vi "Syslog Device Example.vi"() -> ()   [LabVIEW 2016, in "Logger.syslog.lvclass"]
doc: "This VI illustrates sending Syslog debug messages to a collector using the Syslog reference design library."
uses:
  Logger.syslog.lvclass
  <userlib>/_SEH/Controls/CEH/CEH Actions.ctl
  <vilib>/NI/syslog/_subVIs/TypeDefs/syslog_severity_codes.ctl
  <vilib>/NI/syslog/_subVIs/TypeDefs/syslog_facility_codes.ctl
  <userlib>/_OpenG.lib/numeric/numeric.llb/Random Number Within Range - DBL__ogtk.vi
panel:
  out "Waveform Chart":dbl(graph)
  out "Syslog Messages Sent":string
  in  "Collector IP Address":string="0.0.0.0"
  in  "stop":bool
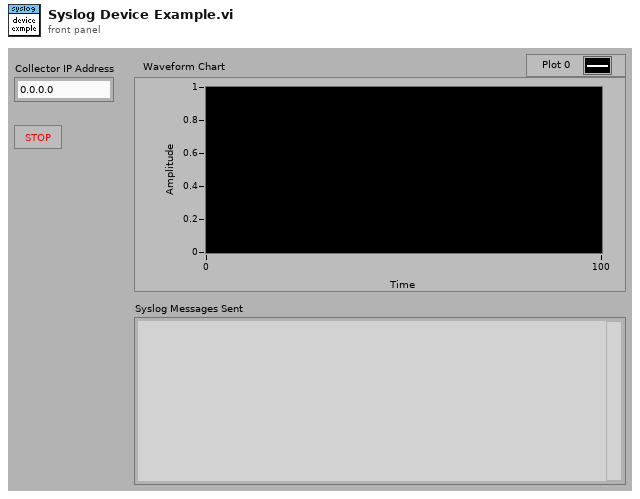
[diagram p1: front panel]
types:
  T1 = typedef "syslog_facility_codes.ctl" = enum16{"kernel", "user", "mail", "system daemons", "security/authorization", "syslogd", "line printer", "network news", "uucp", "clock daemon", "security/authorization (alternate)", "FTP daemon", "NTP subsystem", "log audit", "log alert", "clock daemon (alternate)", "local use 0", "local use 1", "local use 2", "local use 3", "local use 4", "local use 5", "local use 6", "local use 7"}
  T2 = typedef "syslog_severity_codes.ctl" = enum16{"emergency", "alert", "critical", "error", "warning", "notice", "info", "debug"}
  T3 = typedef "CEH Actions.ctl" = enum16{"Log", "Display Error Message", "Safe State", "Shutdown"}
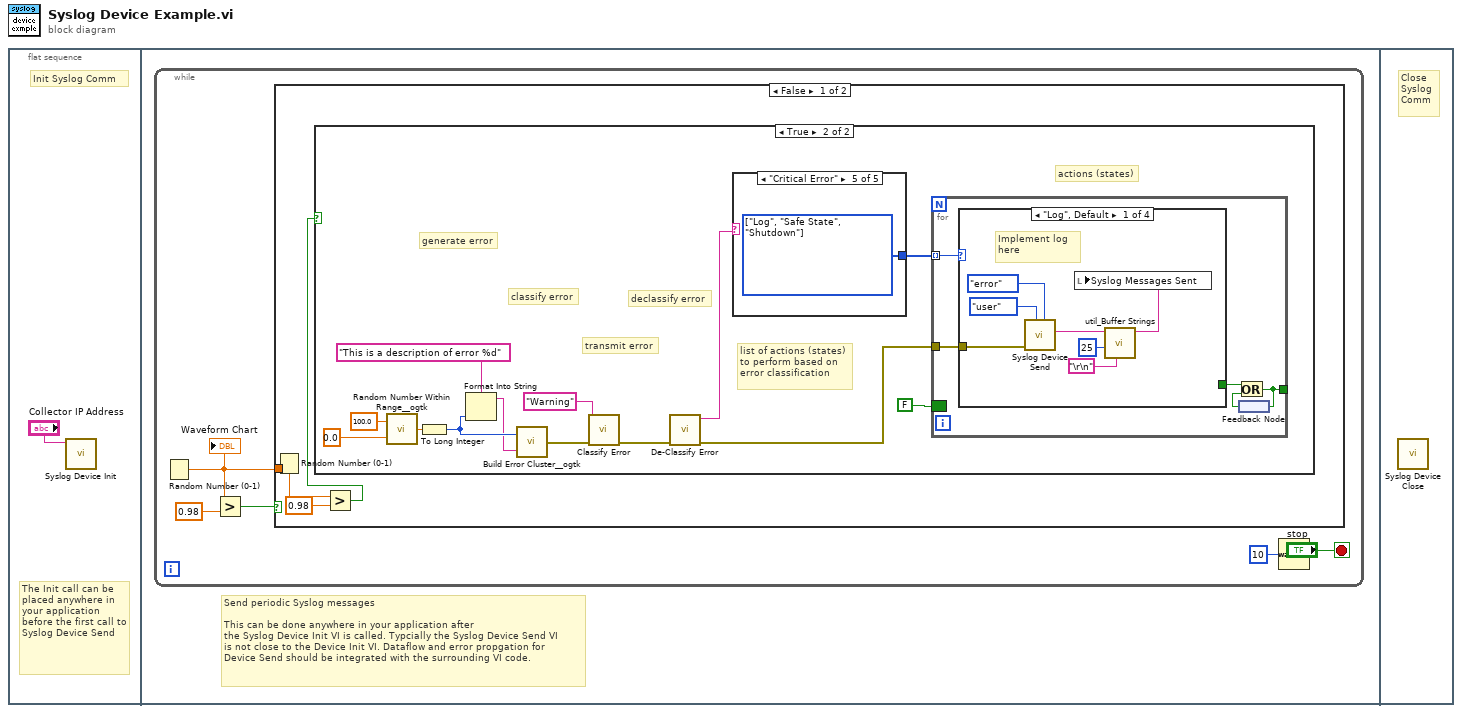
[diagram p0: block diagram]
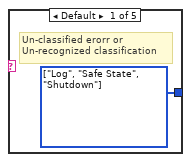
[diagram p3: hidden frame]
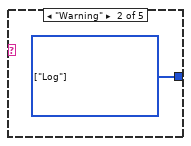
[diagram p4: hidden frame]
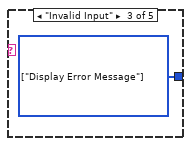
[diagram p5: hidden frame]
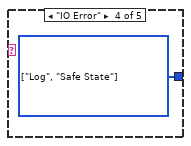
[diagram p6: hidden frame]
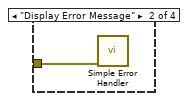
[diagram p7: hidden frame]
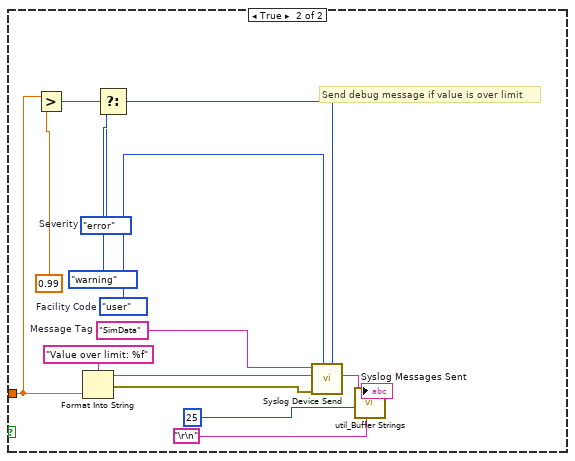
[diagram p10: hidden frame]
diagram:
  n1 = flat-sequence {
    frame #0 {
      # "The Init call can be placed anywhere in your application before the first call to Syslog Device Send"
      # "Init Syslog Comm"
      n2 = call <vilib>:"Syslog Device Init.vi"("Syslog Collector IP Address"="Collector IP Address") -> ()  [unwired: 10 in, 1 out]
    }
    frame #1 {
      # "Send periodic Syslog messages\n\nThis can be done anywhere in your application after\nthe Syslog Device Init VI is called. Typcially the Syslog Device Send VI\nis not close to the Device Init VI. Dataflow and error propgation for \nDevice Send should be integrated with the surrounding VI code."
      n3 = while {
        stop <- "stop" stop-if-true
        n4 = Random Number (0-1)() -> (number: 0 to 1=w2:dbl)
        "Waveform Chart" <- w2
        n5 = Greater?(x=w2, y=0.98) -> (0:w3:bool)
        n6 = case shown="False" w3 {
          tunnel: w2 -> [_ w53]
          frame False {
            n7 = Random Number (0-1)() -> (number: 0 to 1=w9:dbl)
            n8 = Greater?(x=w9, y=0.98) -> (0:w7:bool)
            n9 = case shown="True" w7 {
              frame False {
              }
              frame True {
                # "actions (states)"
                # "list of actions (states)\nto perform based on\nerror classification"
                # "declassify error"
                # "transmit error"
                # "classify error"
                # "generate error"
                n10 = call-poly <userlib>:"Random Number Within Range__ogtk.vi"("High"=100.0, "Low"=0.0) -> ("Random Number"=w19:dbl)  [unwired: 3 in]
                n11 = To Long Integer(number=w19) -> (32bit integer=w18:i32)
                n12 = Format Into String(format string="This is a description of error %d" ("String to Prepend to source (\"\")"), w18) -> (resulting string=w16:string)  [unwired: 2 in, 1 out]
                n13 = call <userlib>:"Build Error Cluster__ogtk.vi"("String to Prepend to source (\"\")"=w16, "code"=w18) -> ("error out"=w17:errorcluster)
                n14 = call <userlib>:"Classify Error.vi"("Error to Classify"=w17, "String"="Warning") -> ("Classified Error"=w13:errorcluster)  [unwired: 9 in]
                n15 = call <userlib>:"De-Classify Error.vi"("Classified Error"=w13) -> ("De-Classified Error"=w10:errorcluster, "Error Classification"=w12:string)  [unwired: 8 in, 1 out]
                n16 = case shown="\"Critical Error\"" w12 {
                  tunnel: [w23 w24 w25 w26 w27] -> w11
                  frame Default {
                    w23 = T3[] [enum."Log", enum."Safe State", enum."Shutdown"] items=["Log", "Display Error Message", "Safe State", "Shutdown"]
                    # "Un-classified erorr or\nUn-recognized classification"
                  }
                  frame "Warning" {
                    w24 = T3[] [enum."Log"] items=["Log", "Display Error Message", "Safe State", "Shutdown"]
                  }
                  frame "Invalid Input" {
                    w25 = T3[] [enum."Display Error Message"] items=["Log", "Display Error Message", "Safe State", "Shutdown"]
                  }
                  frame "IO Error" {
                    w26 = T3[] [enum."Log", enum."Safe State"] items=["Log", "Display Error Message", "Safe State", "Shutdown"]
                  }
                  frame "Critical Error" {
                    w27 = T3[] [enum."Log", enum."Safe State", enum."Shutdown"] items=["Log", "Display Error Message", "Safe State", "Shutdown"]
                  }
                }
                n17 = for {
                  tunnel: w10 -> [w31]
                  tunnel: w11 -> [w32] mode=indexing
                  border: FALSE -> [_]
                  tunnel: [w28] -> _
                  n18 = case shown="\"Log\", Default" w32 {
                    tunnel: w31 -> [w38 w40 _ _]
                    tunnel: [_ _ _ TRUE] -> w30
                    frame "Log", Default {
                      # "Implement log \nhere"
                      n19 = call <vilib>:"Syslog Device Send.vi"("Severity Code (error)"=syslog_severity_codes."error", "Facility Code (user)"=syslog_facility_codes."user", "error in (no error)"=w38) -> ("Syslog Message"=w34:string)  [unwired: 7 in, 1 out]
                      n20 = call <vilib>:"util_Buffer Strings.vi"("Insert between Strings (\"\")"="\r\n", "Number of Strings to Buffer"=u8 25, "New String"=w34) -> ("Buffered String Series"=w33:string)  [unwired: 8 in]
                      n21 = local write "Syslog Messages Sent"(w33) -> ()
                    }
                    frame "Display Error Message" {
                      n22 = call <vilib>:"Simple Error Handler.vi"("error in (no error)"=w40) -> ()  [unwired: 4 in, 5 out]
                    }
                    frame "Safe State" {
                      # "Implement safe\nstate here"
                    }
                    frame "Shutdown" {
                      # "Implement\nshutdown here"
                    }
                  }
                  n23 = feedback #1() -> (w29:bool)
                  n24 = Or(x=w30, y=w29) -> (x .or. y?=w28:bool)
                  n25 = feedback-in #1(w28) -> ()
                }
              }
            }
          }
          frame True {
            w42 = "SimData"  # Message Tag
            w50 = syslog_severity_codes."error"  # Severity
            w56 = syslog_facility_codes."user"  # Facility Code
            # "Send debug message if value is over limit"
            n26 = Greater?(x=w53, y=0.99) -> (0:w52:bool)
            n27 = Format Into String(format string="Value over limit: %f", w53) -> (resulting string=w45:string, error out=w48:errorcluster)  [unwired: 2 in]
            n28 = Select(t=w50, s=w52, f=syslog_severity_codes."warning" ("Severity (error)")) -> (s? t:f=w49:T2)
            n29 = call <vilib>:"Syslog Device Send.vi"("Severity Code (error)"=w49, "Facility Code (user)"=w56, "error in (no error)"=w48, "Message Content"=w45, "Message Tag"=w42) -> ("Syslog Message"=w44:string)  [unwired: 5 in, 1 out]
            n30 = call <vilib>:"util_Buffer Strings.vi"("Insert between Strings (\"\")"="\r\n", "Number of Strings to Buffer"=u8 25, "New String"=w44) -> ("Buffered String Series"=→"Syslog Messages Sent":string)  [unwired: 8 in]
          }
        }
        n31 = Wait (ms)(milliseconds to wait=u32 10 ("millisecond multiple")) -> ()  [unwired: 1 out]
      }
    }
    frame #2 {
      # "Close\nSyslog\nComm"
      n32 = call <vilib>:"Syslog Device Close.vi"() -> ()  [unwired: 11 in, 1 out]
    }
  }
